vi "Command Interpreter.vi"(8 "error in":errorcluster, 11 "Command":string) -> (0 "error out":errorcluster)   [LabVIEW 2014]
doc: "Interprets all incoming commands and takes the appropriate actions."
uses:
  Controls/Switch Program.ctl
  Controls/Action Enum.ctl
  Controls/Switch Day.ctl
  Controls/Switch Schedule FGV.ctl
  Controls/Switch Schedule.ctl
  <vilib>/nisyscfg/Close (System).vi
  <vilib>/nisyscfg/nisyscfg.lvlib
panel:
  out "output cluster":T1
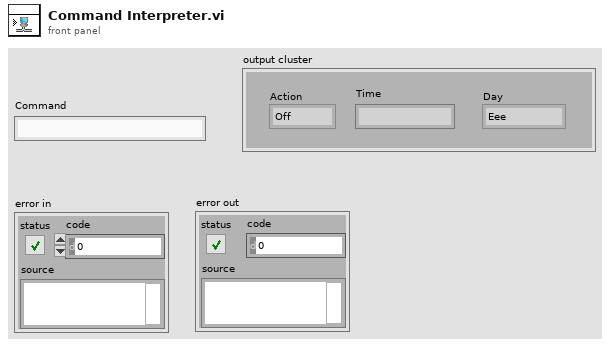
[diagram p1: front panel]
types:
  T1 = typedef "Switch Program.ctl" = cluster{"Action":T2, "Time":string, "Day":T3}
  T2 = typedef "Action Enum.ctl" = enum16{"Off", "On"}
  T3 = typedef "Switch Day.ctl" = enum16{"Eee", "Sun", "Mon", "Tue", "Wed", "Thu", "Fri", "Sat"}
  T4 = typedef "Switch Schedule FGV.ctl" = enum16{"Add", "Delete", "Set", "Get", "Load", "Clear"}
  T5 = typedef "Switch Schedule.ctl" = T1[]
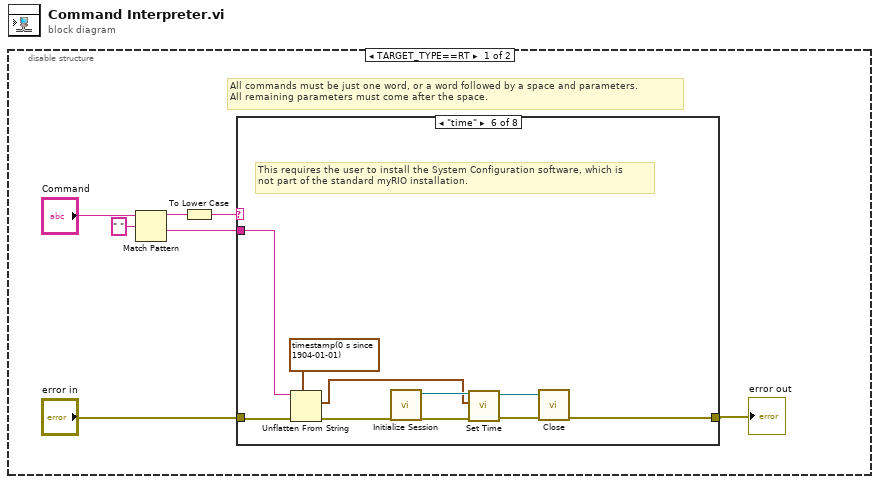
[diagram p0: block diagram]
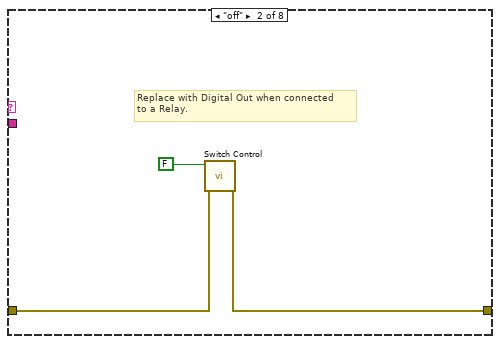
[diagram p3: hidden frame]
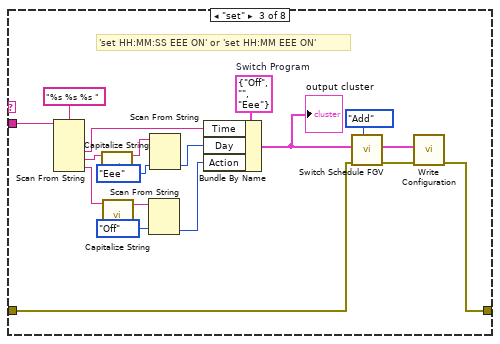
[diagram p4: hidden frame]
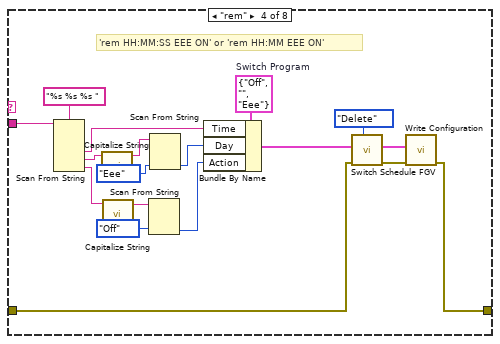
[diagram p5: hidden frame]
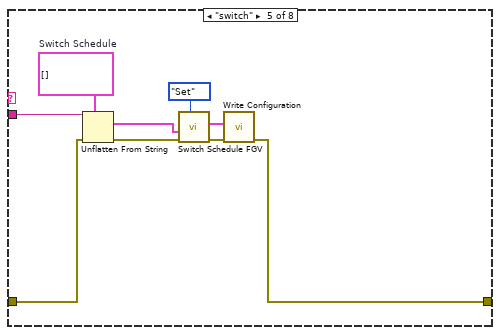
[diagram p6: hidden frame]
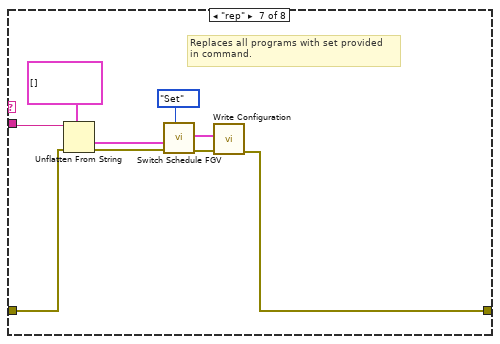
[diagram p7: hidden frame]
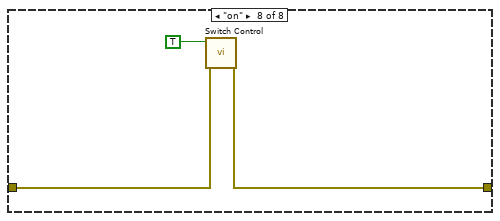
[diagram p8: hidden frame]
diagram:
  n1 = disable-structure shown="TARGET_TYPE==RT" {
    frame condition #0 (active) {
      # "All commands must be just one word, or a word followed by a space and parameters. \nAll remaining parameters must come after the space."
      n2 = Match Pattern(string="Command", regular expression=" ") -> (before substring=w4:string, after substring=w2:string)  [unwired: 1 in, 2 out]
      n3 = To Lower Case(string=w4) -> (all lower case string=w5:string)
      n4 = case shown="\"time\"" w5 {
        tunnel: "error in" -> [w8 w10 w15 w31 w51 w61 w70 w77]
        tunnel: [w8 w11 w13 w30 w48 w62 w67 w76] -> w1
        tunnel: w2 -> [_ _ w29 w47 w56 w59 w75 _]
        frame "False", Default {
        }
        frame "off" {
          # "Replace with Digital Out when connected\nto a Relay."
          n5 = call "Switch Control.vi"("error in (no error)"=w10, "On/Off"=FALSE ("LED0")) -> ("error out"=w11:errorcluster)  [unwired: 9 in]
        }
        frame "set" {
          w25 = T1 {"Action"=enum."Off", "Time"="", "Day"=enum."Eee"}  # Switch Program
          # "'set HH:MM:SS EEE ON' or 'set HH:MM EEE ON'"
          n6 = Scan From String(format string="%s %s %s ", input string=w29) -> (output 1=w24:string, output 2=w21:string, output 3=w18:string)  [unwired: 5 in, 3 out]
          n7 = call "Capitalize String.vi"("String"=w21) -> ("Capitalized String"=w20:string)  [unwired: 10 in]
          n8 = call "Capitalize String.vi"("String"=w18) -> ("Capitalized String"=w19:string)  [unwired: 10 in]
          n9 = Scan From String(input string=w19, default 1=Action_Enum."Off" ("Action")) -> (output 1=w22:T2)  [unwired: 3 in, 3 out]
          n10 = Scan From String(input string=w20, default 1=Switch_Day."Eee" ("Day")) -> (output 1=w23:T3)  [unwired: 3 in, 3 out]
          n11 = Bundle By Name(cluster=w25, "Time"=w24, "Day"=w23, "Action"=w22) -> (w17:T1)
          "output cluster" <- w17
          n12 = call "Switch Schedule FGV.vi"("Action"=Switch_Schedule_FGV."Add", "error in (no error)"=w15, "Switch Program"=w17) -> ("error out"=w14:errorcluster, "Switch Schedule"=w12:T5)  [unwired: 7 in]
          n13 = call "Write Configuration.vi"("error in (no error)"=w14, "Switch Schedule"=w12) -> ("error out"=w13:errorcluster)  [unwired: 9 in]
        }
        frame "rem" {
          w43 = T1 {"Action"=enum."Off", "Time"="", "Day"=enum."Eee"}  # Switch Program
          # "'rem HH:MM:SS EEE ON' or 'rem HH:MM EEE ON'"
          n14 = Scan From String(format string="%s %s %s ", input string=w47) -> (output 1=w42:string, output 2=w39:string, output 3=w36:string)  [unwired: 5 in, 3 out]
          n15 = call "Capitalize String.vi"("String"=w39) -> ("Capitalized String"=w38:string)  [unwired: 10 in]
          n16 = call "Capitalize String.vi"("String"=w36) -> ("Capitalized String"=w37:string)  [unwired: 10 in]
          n17 = Scan From String(input string=w37, default 1=Action_Enum."Off" ("Action")) -> (output 1=w40:T2)  [unwired: 3 in, 3 out]
          n18 = Scan From String(input string=w38, default 1=Switch_Day."Eee" ("Day")) -> (output 1=w41:T3)  [unwired: 3 in, 3 out]
          n19 = Bundle By Name(cluster=w43, "Time"=w42, "Day"=w41, "Action"=w40) -> (w35:T1)
          n20 = call "Switch Schedule FGV.vi"("Action"=Switch_Schedule_FGV."Delete", "error in (no error)"=w31, "Switch Program"=w35) -> ("error out"=w33:errorcluster, "Switch Schedule"=w32:T5)  [unwired: 7 in]
          n21 = call "Write Configuration.vi"("error in (no error)"=w33, "Switch Schedule"=w32) -> ("error out"=w30:errorcluster)  [unwired: 9 in]
        }
        frame "switch" {
          w55 = T5 []  # Switch Schedule
          n22 = Unflatten From String(type=w55, binary string=w56, error in (no error)=w51) -> (value=w53:T5, error out=w54:errorcluster)  [unwired: 2 in, 1 out]
          n23 = call "Switch Schedule FGV.vi"("Action"=Switch_Schedule_FGV."Set", "error in (no error)"=w54, "Switch Schedule"=w53) -> ("error out"=w50:errorcluster, "Switch Schedule"=w49:T5)  [unwired: 7 in]
          n24 = call "Write Configuration.vi"("error in (no error)"=w50, "Switch Schedule"=w49) -> ("error out"=w48:errorcluster)  [unwired: 9 in]
        }
        frame "time" {
          # "This requires the user to install the System Configuration software, which is\nnot part of the standard myRIO installation."
          n25 = Unflatten From String(type=timestamp(0 s since 1904-01-01) ("Time Stamp"), binary string=w59, error in (no error)=w61) -> (value=w57:timestamp, error out=w60:errorcluster)  [unwired: 2 in, 1 out]
          n26 = call <vilib>:"Initialize Session.vi"("error in (no error)"=w60) -> ("error out"=w65:errorcluster, "Session out"=w66:refnum<k21>)  [unwired: 9 in]
          n27 = call <vilib>:"Set Time.vi"("error in (no error)"=w65, "Time"=w57, "Session in (localhost)"=w66) -> ("error out"=w63:errorcluster, "Session out"=w64:refnum<k21>)  [unwired: 5 in, 2 out]
          n28 = call-poly <vilib>:"Close.vi"("error in (no error)"=w63, "Session in"=w64) -> ("error out"=w62:errorcluster)  [unwired: 9 in]
        }
        frame "rep" {
          # "Replaces all programs with set provided\nin command."
          n29 = Unflatten From String(type=T5 [] ("Switch Schedule"), binary string=w75, error in (no error)=w70) -> (value=w71:T5, error out=w73:errorcluster)  [unwired: 2 in, 1 out]
          n30 = call "Switch Schedule FGV.vi"("Action"=Switch_Schedule_FGV."Set", "error in (no error)"=w73, "Switch Schedule"=w71) -> ("error out"=w69:errorcluster, "Switch Schedule"=w68:T5)  [unwired: 7 in]
          n31 = call "Write Configuration.vi"("error in (no error)"=w69, "Switch Schedule"=w68) -> ("error out"=w67:errorcluster)  [unwired: 9 in]
        }
        frame "on" {
          n32 = call "Switch Control.vi"("error in (no error)"=w77, "On/Off"=TRUE ("LED0")) -> ("error out"=w76:errorcluster)  [unwired: 9 in]
        }
      }
      "error out" <- w1
    }
    frame condition #1 {
    }
  }
